vi "Kinect Override or Normal.vi"(11 "KinectEnabled?":bool) -> ()   [LabVIEW 2011]
uses:
  Team Code/Robot Global Data.vi
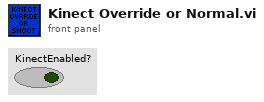
[diagram p1: front panel]
types:
  T1 = cluster{"Left Arm":dbl, "Right Arm":dbl, "Head Right":bool, "Head Left":bool, "Right Leg to Right":bool, "Left Leg to Left":bool, "Right Leg Forward":bool, "Right Leg Back":bool, "Left Leg Forward":bool, "Left Leg Back":bool, "Enable":bool, "Distance":dbl, "Enable Override?":bool, "FIRE!!!!":bool}
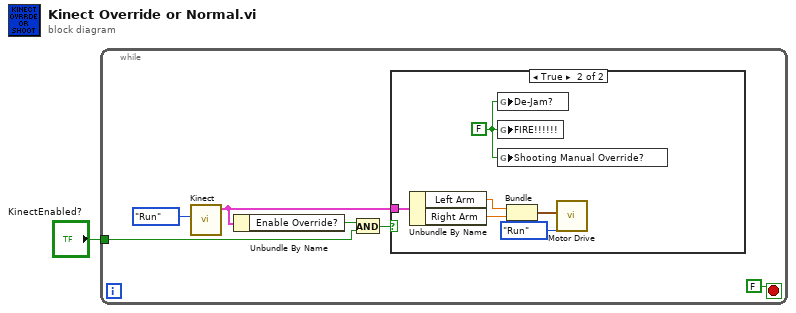
[diagram p0: block diagram]
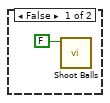
[diagram p2: hidden frame]
diagram:
  n1 = while {
    tunnel: "KinectEnabled?" -> [w4]
    stop <- FALSE stop-if-true
    n2 = call "Kinect.vi"("Mode"=enum16{"Init", "Run", "End"}."Run") -> ("Kinect"=w2:T1)  [unwired: 10 in]
    n3 = Unbundle By Name(w2) -> ("Enable Override?"=w5:bool)
    n4 = And(x=w5, y=w4) -> (x .and. y?=w3:bool)
    n5 = case shown="True" w3 {
      tunnel: w2 -> [_ w14]
      frame False {
        n6 = call "Shoot Balls.vi"("Use Kinect?"=FALSE) -> ()  [unwired: 10 in, 1 out]
      }
      frame True {
        w10 = FALSE ("De-Jam?")
        n7 = Unbundle By Name(w14) -> ("Left Arm"=w12:dbl, "Right Arm"=w11:dbl)
        n8 = global write "Robot Global Data.vi" "De-Jam?"(w10) -> ()
        n9 = global write "Robot Global Data.vi" "FIRE!!!!!!"(w10) -> ()
        n10 = global write "Robot Global Data.vi" "Shooting Manual Override?"(w10) -> ()
        n11 = Bundle("Left Arm"=w12, "Right Arm"=w11) -> (w13:cluster{"Left Arm":dbl, "Right Arm":dbl})  [unwired: 1 in]
        n12 = call "Motor Drive.vi"("Motor Input"=w13, "Enum"=enum16{"Init", "Run", "SetBrakeCoast", "End"}."Run") -> ()  [unwired: 10 in]
      }
    }
  }
